vi "Morphological Segmentation Example.vi"() -> ()   [LabVIEW 2011]
doc: "This example demonstrates a watershed transform as part of a morphological segmentation process. First, a sample image is thesholded, and a distance transform is applied to the sample image. Next, a watershed transform is applied to the image. The resulting watershed lines appear in a different color to show how the watershed transform separated touching objects and segmented the image."
uses:
  <vilib>/vision/NI_Vision_Development_Module.lvlib
panel:
  in  "Sample Image":path
  in  "Connectivity 8":bool=TRUE
  out "Image":T1(plugin-control) caption="Sample Image"
  in  "Stop":bool
  in  "Run Current Step":bool
  out "Morphological Segmentation Steps":i32(listbox)=6
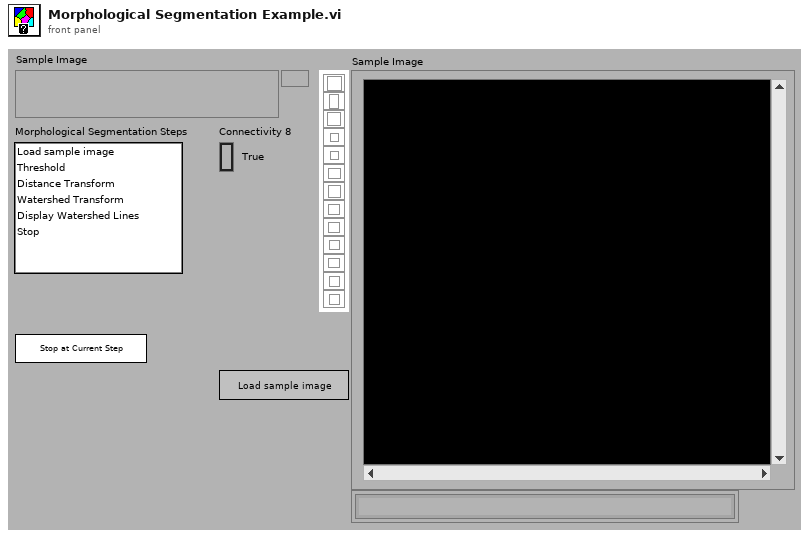
[diagram p1: front panel]
types:
  T1 = typedef "IMAQ Image.ctl" = refnum<image>
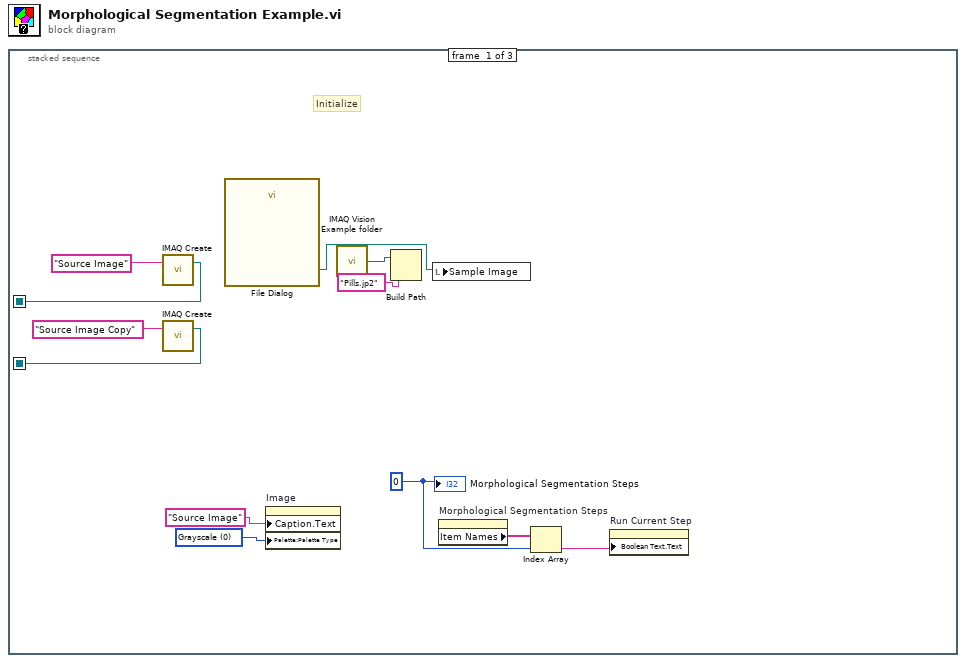
[diagram p0: block diagram]
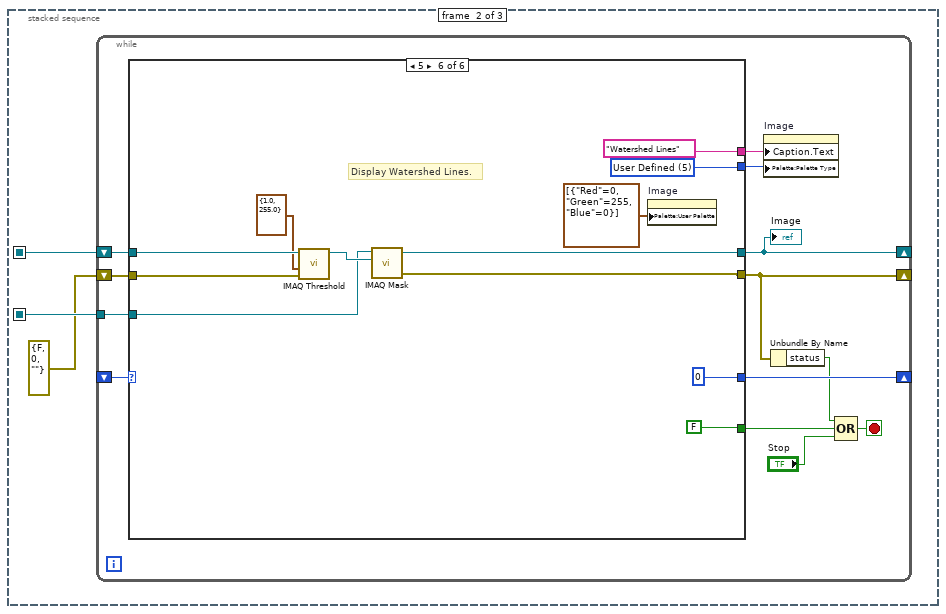
[diagram p2: hidden frame]
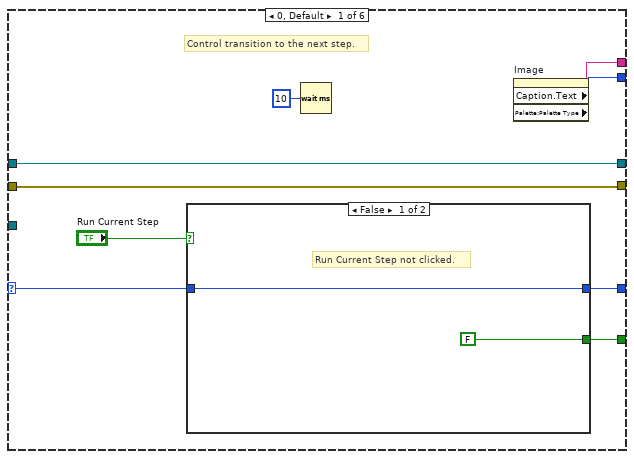
[diagram p3: hidden frame]
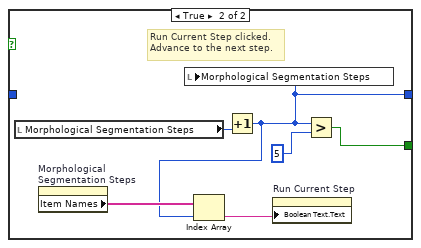
[diagram p4: hidden frame]
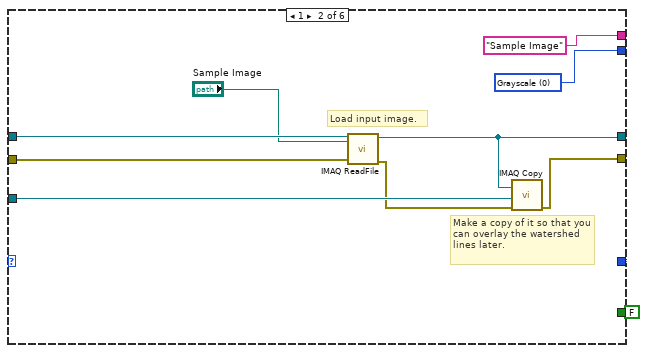
[diagram p5: hidden frame]
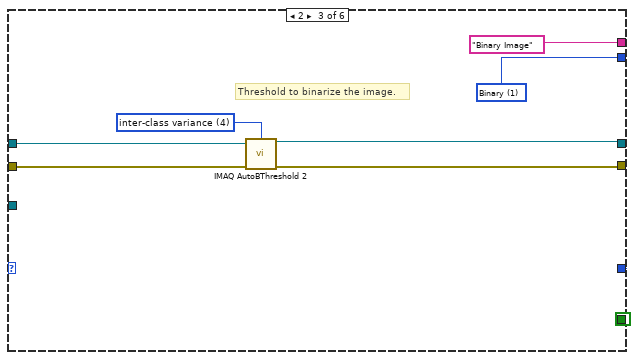
[diagram p6: hidden frame]
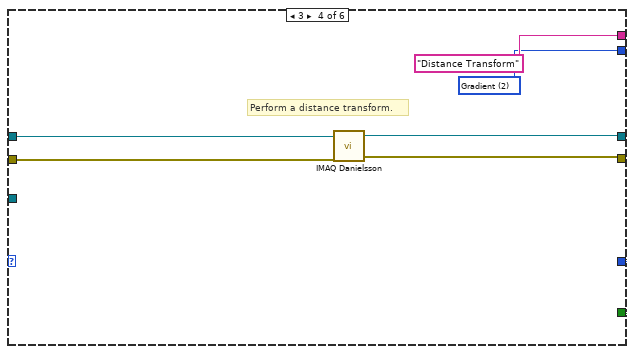
[diagram p7: hidden frame]
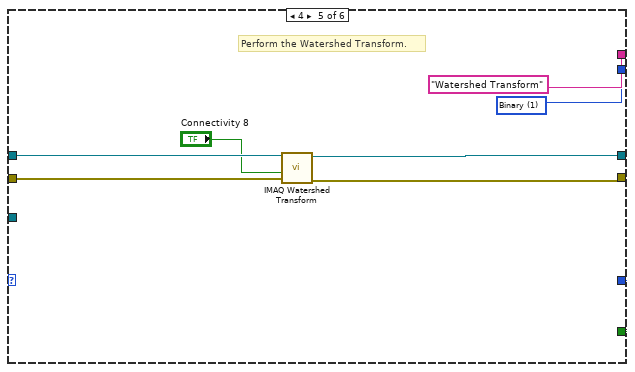
[diagram p8: hidden frame]
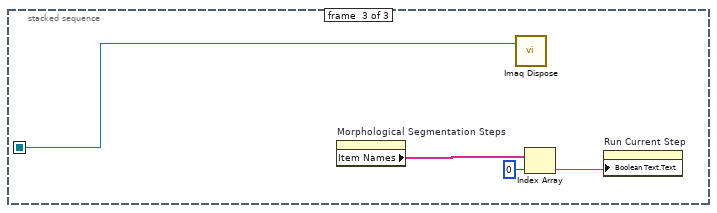
[diagram p9: hidden frame]
diagram:
  n1 = stacked-sequence {
    seq-local: [w8 _ _] -> [_ w14 w95]
    seq-local: [w7 _ _] -> [_ w15 _]
    frame #0 {
      w10 = u32 0 items=["Grayscale", "Binary", "Gradient", "Rainbow", "Temperature", "User Defined"] ("Palette:Palette Type")
      w4 = 0
      # "Initialize"
      n2 = call "IMAQ Create"("Image Name"="Source Image") -> ("New Image"=w8:T1)  [unwired: 3 in, 2 out]
      n3 = call "IMAQ Create"("Image Name"="Source Image Copy") -> ("New Image"=w7:T1)  [unwired: 3 in, 2 out]
      n4 = call "File Dialog"() -> ("selected path"=w1:path)  [unwired: 12 in, 3 out]
      n5 = property on="Image" class="ImageControl"("Caption.Text"="Source Image", "Palette:Palette Type"=w10) -> ()  [unwired: 2 in, 2 out]
      n6 = call "IMAQ Vision Example folder.vi"() -> ("Example Image Path"=w2:path)  [unwired: 1 out]
      n7 = Build Path(base path=w2, name or relative path="Pills.jp2") -> ()  [unwired: 1 out]
      n8 = local write "Sample Image"(w1) -> ()
      n9 = property on="Morphological Segmentation Steps" class="LstBox (strict)"() -> ("Item Names"=w6:string[])  [unwired: 2 in, 2 out]
      n10 = Index Array(array=w6, index=w4) -> (element=w5:string)
      n11 = property on="Run Current Step" class="Bool"("Boolean Text.Text"=w5) -> ()  [unwired: 2 in, 2 out]
      "Morphological Segmentation Steps" <- w4
    }
    frame #1 {
      n12 = while {
        shift-right: [w24] -> _
        shift-left: _ -> [w25]
        tunnel: w15 -> [w18]
        shift-right: [w19] -> _
        shift-left: errorcluster {"status"=FALSE, "code"=0, "source"=""} ("error out") -> [w16]
        shift-right: [w17] -> _
        shift-left: w14 -> [w28]
        stop <- w27 stop-if-true
        n13 = case shown="5" w25 {
          selector: w25 -> [w36 _ _ _ _ _]
          tunnel: w28 -> [w35 w52 w57 w69 w77 w90]
          tunnel: [w29 w49 w58 w67 w78 w83] -> w19
          tunnel: [w30 0 0 0 0 0] -> w24
          tunnel: [w34 "Sample Image" ("Title") "Binary Image" ("Title") "Distance Transform" ("Title") "Watershed Transform" ("Title") "Watershed Lines" ("Title")] -> w22
          tunnel: [w33 w54 w62 w71 w80 w91] -> w23
          tunnel: [w32 FALSE FALSE FALSE FALSE FALSE] -> w20
          tunnel: w18 -> [_ w53 _ _ _ w86]
          tunnel: [w35 w51 w59 w68 w75 w85] -> w17
          tunnel: w16 -> [w29 w47 w60 w66 w74 w89]
          frame 0, Default {
            # "Control transition to the next step."
            n14 = case shown="False" "Run Current Step" {
              tunnel: w36 -> [w38 _]
              tunnel: [FALSE w44] -> w32
              tunnel: [w38 w40] -> w30
              frame False {
                # "Run Current Step not clicked."
              }
              frame True {
                # "Run Current Step clicked.\nAdvance to the next step."
                n15 = local read "Morphological Segmentation Steps"() -> (w42:i32)
                n16 = property on="Morphological Segmentation Steps" class="LstBox (strict)"() -> ("Item Names"=w43:string[])  [unwired: 2 in, 2 out]
                n17 = Increment(x=w42) -> (x+1=w40:i32)
                n18 = local write "Morphological Segmentation Steps"(w40) -> ()
                n19 = Index Array(array=w43, index=w40) -> (element=w41:string)
                n20 = property on="Run Current Step" class="Bool"("Boolean Text.Text"=w41) -> ()  [unwired: 2 in, 2 out]
                n21 = Greater?(x=w40, y=5) -> (0:w44:bool)
              }
            }
            n22 = Wait (ms)(milliseconds to wait=u32 10) -> ()  [unwired: 1 out]
            n23 = property on="Image" class="ImageControl"() -> ("Caption.Text"=w34:string, "Palette:Palette Type"=w33:u32)  [unwired: 2 in, 2 out]
          }
          frame 1 {
            w54 = u32 0 items=["Grayscale", "Binary", "Gradient", "Rainbow", "Temperature", "User Defined"] ("Palette:Palette Type")
            # "Make a copy of it so that you can overlay the watershed lines later."
            # "Load input image."
            n24 = call "IMAQ ReadFile"("File Path"="Sample Image", "error in (no error)"=w47, "Image"=w52) -> ("error out"=w50:errorcluster, "Image Out"=w51:T1)  [unwired: 2 in, 5 out]
            n25 = call "IMAQ Copy"("error in (no error)"=w50, "Image Dst"=w53, "Image Src"=w51) -> ("error out"=w49:errorcluster)  [unwired: 4 out]
          }
          frame 2 {
            w61 = 4 items=["clustering", "entropy", "metric", "moments", "inter-class variance"] ("Method")
            w62 = u32 1 items=["Grayscale", "Binary", "Gradient", "Rainbow", "Temperature", "User Defined"] ("Palette:Palette Type")
            # "Threshold to binarize the image."
            n26 = call "IMAQ AutoBThreshold 2"("Image Src"=w57, "Method (clustering)"=w61, "error in (no error)"=w60) -> ("Image Dst Out"=w59:T1, "error out"=w58:errorcluster)  [unwired: 5 in, 6 out]
          }
          frame 3 {
            w71 = u32 2 items=["Grayscale", "Binary", "Gradient", "Rainbow", "Temperature", "User Defined"] ("Palette:Palette Type")
            # "Perform a distance transform."
            n27 = call "IMAQ Danielsson"("error in (no error)"=w66, "Image Src"=w69) -> ("error out"=w67:errorcluster, "Image Dst Out"=w68:T1)  [unwired: 1 in, 1 out]
          }
          frame 4 {
            w80 = u32 1 items=["Grayscale", "Binary", "Gradient", "Rainbow", "Temperature", "User Defined"] ("Palette:Palette Type")
            # "Perform the Watershed Transform."
            n28 = call "IMAQ Watershed Transform"("error in (no error)"=w74, "Connectivity 4/8 (8)"="Connectivity 8", "Image Src"=w77) -> ("error out"=w78:errorcluster, "Image Dst Out"=w75:T1)  [unwired: 1 in, 6 out]
          }
          frame 5 {
            w91 = u32 5 items=["Grayscale", "Binary", "Gradient", "Rainbow", "Temperature", "User Defined"] ("Palette:Palette Type")
            # "Display Watershed Lines."
            n29 = call "IMAQ Threshold"("error in (no error)"=w89, "Range"=cluster{"Lower value":sgl, "Upper value":sgl} {"Lower value"=1.0, "Upper value"=255.0}, "Image Src"=w90) -> ("Image Dst Out"=w87:T1)  [unwired: 3 in, 5 out]
            n30 = call "IMAQ Mask"("Image Mask"=w87, "Image Src"=w86) -> ("error out"=w83:errorcluster, "Image Dst Out"=w85:T1)  [unwired: 2 in, 1 out]
            n31 = property on="Image" class="ImageControl"("Palette:User Palette"=cluster{"Red":u8, "Green":u8, "Blue":u8}[] [{"Red"=0, "Green"=255, "Blue"=0}]) -> ()  [unwired: 2 in, 2 out]
          }
        }
        "Image" <- w17
        n32 = property on="Image" class="ImageControl"("Caption.Text"=w22, "Palette:Palette Type"=w23) -> ()  [unwired: 2 in, 2 out]
        n33 = Unbundle By Name(w19) -> ("status"=w21:bool)
        n34 = Compound Arithmetic op=OR(w21, w20, "Stop") -> (w27:bool)
      }
    }
    frame #2 {
      n35 = property on="Morphological Segmentation Steps" class="LstBox (strict)"() -> ("Item Names"=w98:string[])  [unwired: 2 in, 2 out]
      n36 = call "Imaq Dispose"("Image"=w95) -> ()  [unwired: 2 in, 4 out]
      n37 = Index Array(array=w98, index=0) -> (element=w97:string)
      n38 = property on="Run Current Step" class="Bool"("Boolean Text.Text"=w97) -> ()  [unwired: 2 in, 2 out]
    }
  }
